vi "Read All Inputs.vi"(8 "error in":errorcluster, 10 "Voltage":bool=TRUE, 11 "VISA resource name":refnum<visa-resource-name>) -> (0 "error out":errorcluster, 1 "Digital Output cluster":T1, 2 "Analog output cluster":T2, 3 "VISA resource name out":refnum<visa-resource-name>)   [LabVIEW 2020, in "BDAQ-6104.lvlib"]
uses:
  <instrlib>/BDAQ-6104/BDAQ-6104.lvlib
panel:
  in  "DIO CLuster":T1
  out "Volts 5":dbl
  out "Volts 4":dbl
  out "Volts 3":dbl
  out "Volts 2":dbl
  out "Volts 1":dbl
  out "Volts 0":dbl
  out "Value 5":i32
  out "Value 4":i32
  out "Value 3":i32
  out "Vaolue 2":i32
  out "Value 1":i32
  out "Value 0":i32
  out "Bytes Read":u32
  in  "AIO Cluster":T2
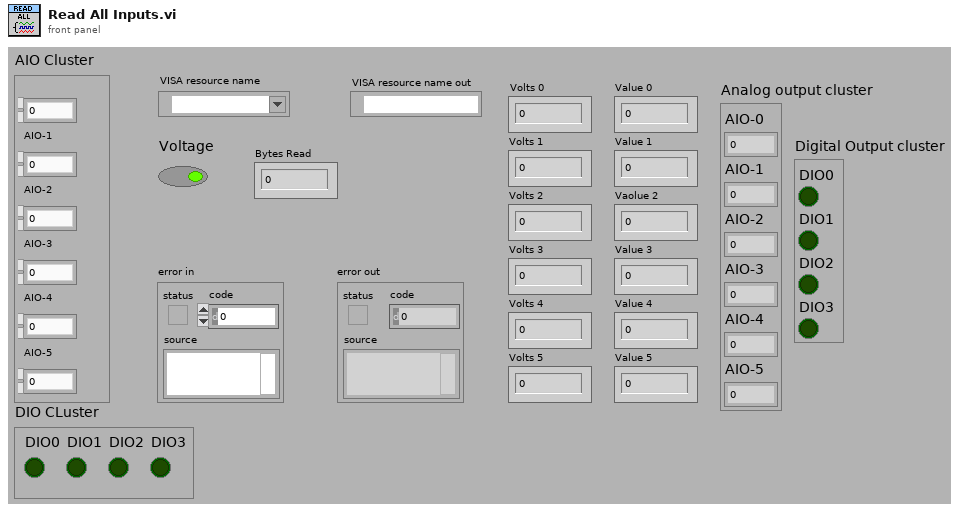
[diagram p1: front panel]
types:
  T1 = cluster{"DIO0":bool, "DIO2":bool, "DIO3":bool, "DIO1":bool}
  T2 = cluster{"AIO-0":dbl, "AIO-1":dbl, "AIO-2":dbl, "AIO-3":dbl, "AIO-4":dbl, "AIO-5":dbl}
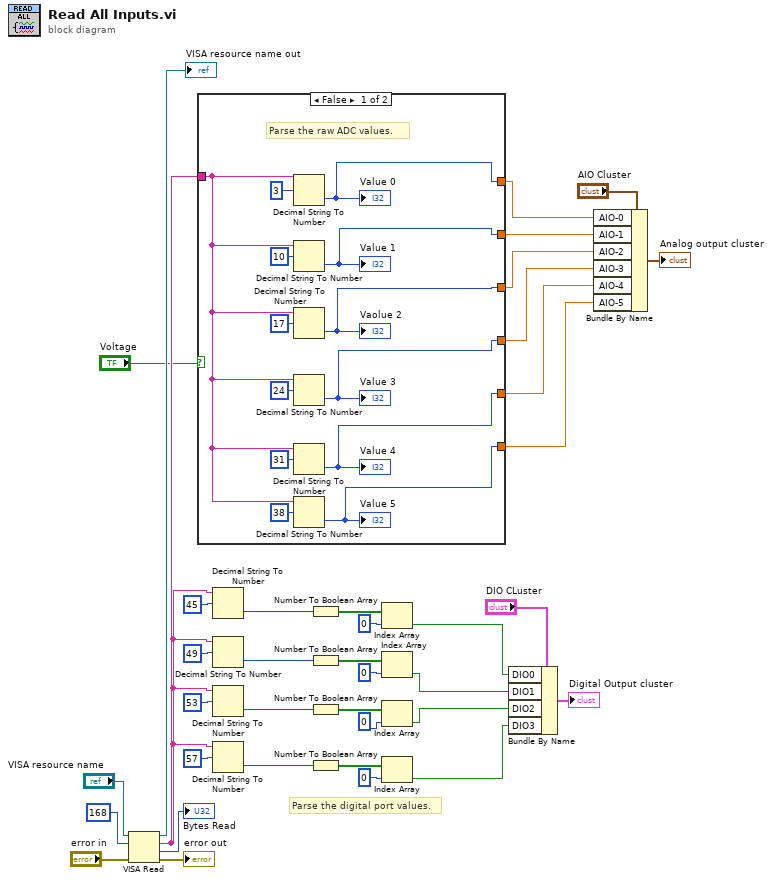
[diagram p0: block diagram]
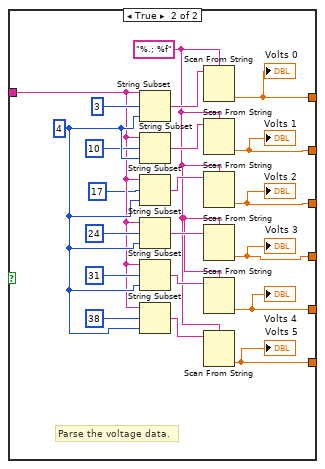
[diagram p2: hidden frame]
diagram:
  # "Parse the digital port values."
  n1 = VISA Read(VISA resource name="VISA resource name", byte count=u32 168, error in (no error)="error in") -> (VISA resource name out=→"VISA resource name out":refnum<visa-resource-name>, read buffer=w15:string, return count=→"Bytes Read":u32, error out=→"error out":errorcluster)
  n2 = case shown="False" "Voltage" {
    tunnel: w15 -> [w45 w66]
    tunnel: [w44 w58] -> w13
    tunnel: [w43 w57] -> w12
    tunnel: [w42 w56] -> w11
    tunnel: [w41 w55] -> w10
    tunnel: [w40 w54] -> w9
    tunnel: [w39 w53] -> w8
    frame False {
      # "Parse the raw ADC values."
      n3 = Decimal String To Number(string=w45, offset=3) -> (number=w44:i32)  [unwired: 1 in, 1 out]
      "Value 0" <- w44
      n4 = Decimal String To Number(string=w45, offset=10) -> (number=w43:i32)  [unwired: 1 in, 1 out]
      "Value 1" <- w43
      n5 = Decimal String To Number(string=w45, offset=17) -> (number=w42:i32)  [unwired: 1 in, 1 out]
      "Vaolue 2" <- w42
      n6 = Decimal String To Number(string=w45, offset=24) -> (number=w41:i32)  [unwired: 1 in, 1 out]
      "Value 3" <- w41
      n7 = Decimal String To Number(string=w45, offset=31) -> (number=w40:i32)  [unwired: 1 in, 1 out]
      "Value 4" <- w40
      n8 = Decimal String To Number(string=w45, offset=38) -> (number=w39:i32)  [unwired: 1 in, 1 out]
      "Value 5" <- w39
    }
    frame True {
      w59 = "%.; %f" ("format string")
      w71 = 4 ("length (rest)")
      # "Parse the voltage data."
      n9 = String Subset(string=w66, offset (0)=3, length (rest)=w71) -> (substring=w65:string)
      n10 = String Subset(string=w66, offset (0)=10, length (rest)=w71) -> (substring=w64:string)
      n11 = String Subset(string=w66, offset (0)=17 ("length (rest)"), length (rest)=w71) -> (substring=w63:string)
      n12 = String Subset(string=w66, offset (0)=24, length (rest)=w71) -> (substring=w62:string)
      n13 = String Subset(string=w66, offset (0)=31, length (rest)=w71) -> (substring=w61:string)
      n14 = String Subset(string=w66, offset (0)=38, length (rest)=w71) -> (substring=w60:string)
      n15 = Scan From String(format string=w59, input string=w65) -> (output 1=w58:dbl)  [unwired: 3 in, 3 out]
      "Volts 0" <- w58
      n16 = Scan From String(format string=w59, input string=w64) -> (output 1=w57:dbl)  [unwired: 3 in, 3 out]
      "Volts 1" <- w57
      n17 = Scan From String(format string=w59, input string=w63) -> (output 1=w56:dbl)  [unwired: 3 in, 3 out]
      "Volts 2" <- w56
      n18 = Scan From String(format string=w59, input string=w62) -> (output 1=w55:dbl)  [unwired: 3 in, 3 out]
      "Volts 3" <- w55
      n19 = Scan From String(format string=w59, input string=w61) -> (output 1=w54:dbl)  [unwired: 3 in, 3 out]
      "Volts 4" <- w54
      n20 = Scan From String(format string=w59, input string=w60) -> (output 1=w53:dbl)  [unwired: 3 in, 3 out]
      "Volts 5" <- w53
    }
  }
  n21 = Decimal String To Number(string=w15, offset=45) -> (number=w35:i32)  [unwired: 1 in, 1 out]
  n22 = Decimal String To Number(string=w15, offset=49) -> (number=w31:i32)  [unwired: 1 in, 1 out]
  n23 = Decimal String To Number(string=w15, offset=53) -> (number=w27:i32)  [unwired: 1 in, 1 out]
  n24 = Decimal String To Number(string=w15, offset=57) -> (number=w23:i32)  [unwired: 1 in, 1 out]
  n25 = Number To Boolean Array(number=w35) -> (Boolean array=w34:bool[])
  n26 = Number To Boolean Array(number=w31) -> (Boolean array=w30:bool[])
  n27 = Number To Boolean Array(number=w27) -> (Boolean array=w26:bool[])
  n28 = Number To Boolean Array(number=w23) -> (Boolean array=w22:bool[])
  n29 = Index Array(array=w34, index=0) -> (element=w5:bool)
  n30 = Index Array(array=w30, index=0) -> (element=w4:bool)
  n31 = Index Array(array=w26, index=0) -> (element=w3:bool)
  n32 = Index Array(array=w22, index=0) -> (element=w2:bool)
  n33 = Bundle By Name(cluster="DIO CLuster", "DIO0"=w5, "DIO1"=w4, "DIO2"=w3, "DIO3"=w2) -> (→"Digital Output cluster":T1)
  n34 = Bundle By Name(cluster="AIO Cluster", "AIO-0"=w13, "AIO-1"=w12, "AIO-2"=w11, "AIO-3"=w10, "AIO-4"=w9, "AIO-5"=w8) -> (→"Analog output cluster":T2)
